vi "Engine Out - Faults - Oil Temp.vi"(11 "Oil Temp [C]":sgl) -> ()   [LabVIEW 2015, in "ECS-RT.lvlib"]
uses:
  ECS-RT.lvlib
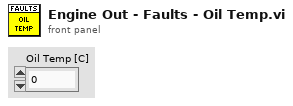
[diagram p1: front panel]
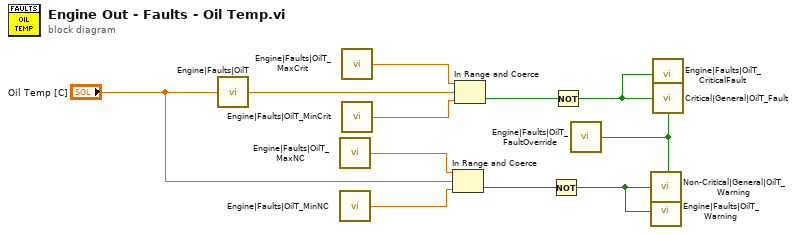
[diagram p0: block diagram]
diagram:
  n1 = call "Engine|Faults|OilT"("Value"="Oil Temp [C]") -> ()
  n2 = call "Engine|Faults|OilT_MaxNC"() -> ("Value"=w7:sgl)
  n3 = call "Engine|Faults|OilT_MinNC"() -> ("Value"=w8:sgl)
  n4 = call "Engine|Faults|OilT_MaxCrit"() -> ("Value"=w3:sgl)
  n5 = call "Engine|Faults|OilT_MinCrit"() -> ("Value"=w4:sgl)
  n6 = In Range and Coerce(upper limit=w7, x="Oil Temp [C]", lower limit=w8) -> (In Range?=w9:bool)  [unwired: 1 out]
  n7 = In Range and Coerce(upper limit=w3, x="Oil Temp [C]", lower limit=w4) -> (In Range?=w5:bool)  [unwired: 1 out]
  n8 = Not(x=w9) -> (.not. x?=w10:bool)
  n9 = Not(x=w5) -> (.not. x?=w6:bool)
  n10 = call "Engine|Faults|OilT_FaultOverride"() -> ("Value"=w1:bool)
  n11 = call "Non-Critical|General|OilT_Warning"("Fault"=w10, "Override (F)"=w1) -> ()  [unwired: 1 in]
  n12 = call "Engine|Faults|OilT_Warning"("Value"=w10) -> ()
  n13 = call "Engine|Faults|OilT_CriticalFault"("Value"=w6) -> ()
  n14 = call "Critical|General|OilT_Fault"("Fault"=w6, "Override (F)"=w1) -> ()  [unwired: 1 in]
